vi "readFromXML.vi"(8 "error in (no error)":errorcluster, 10 "XML in":string, 11 "TCSCommand in":refnum<class "TCSCommand.lvclass">) -> (0 "error out":errorcluster, 3 "TCSCommand out":refnum<class "TCSCommand.lvclass">)   [LabVIEW 2014, in "TCSDataDefinitions.lvlib" / "TCSCommand.lvlib" / "TCSCommand.lvclass"]
uses:
  TCSCommand.lvclass
  TCSCommand.lvclass/TCSCommand.ctl
  <userlib>/Common/XML/XMLParser/XMLParser.lvclass
panel:
  out "tcsErrorResponse":errorcluster
  out "commandID":u32
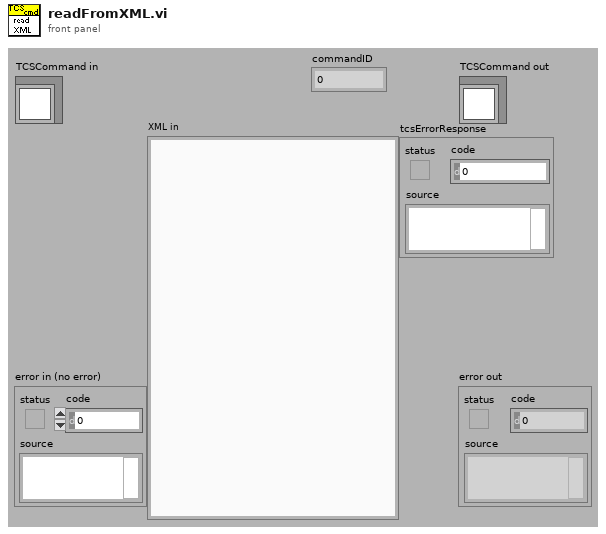
[diagram p1: front panel]
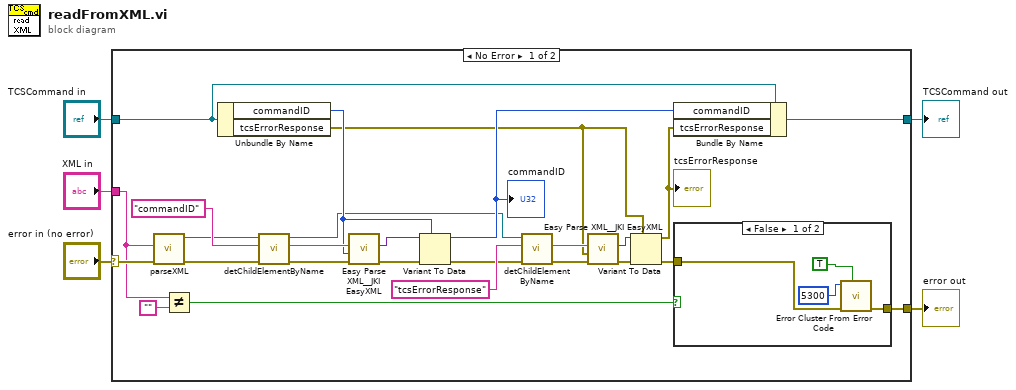
[diagram p0: block diagram]
diagram:
  n1 = case shown="No Error" "error in (no error)" {
    selector: "error in (no error)" -> [w29 w38]
    tunnel: [w10 w38] -> w4
    tunnel: [w15 w37] -> w2
    tunnel: "TCSCommand in" -> [w11 w37]
    tunnel: "XML in" -> [w9 _]
    frame No Error {
      n2 = call <userlib>:"parseXML.vi"("error in (no error)"=w29, "XMLString in"=w9) -> ("error out"=w13:errorcluster, "Element out"=w7:refnum<class "XMLParser.lvclass">)  [unwired: 8 in]
      n3 = Not Equal?(x=w9, y="") -> (x != y?=w30:bool)
      n4 = Unbundle By Name(w11) -> ("commandID"=w21:u32, "tcsErrorResponse"=w12:errorcluster)
      n5 = call <userlib>:"detChildElementByName.vi"("error in (no error)"=w13, "childName"="commandID" ("ChildName"), "Element in"=w7) -> ("error out"=w22:errorcluster, "childXML"=w26:string, "Element out"=w6:refnum<class "XMLParser.lvclass">)  [unwired: 5 in, 1 out]
      n6 = call <vilib>:"Easy Parse XML__JKI EasyXML.vi"("error in (no error)"=w22, "LabVIEW Data (Type)"=w21, "XML String"=w26) -> ("error out"=w23:errorcluster, "LabVIEW Data"=w24:variant)  [unwired: 7 in]
      n7 = Variant To Data(error in=w23, type=w21, Variant=w24) -> (data=w20:u32, error out=w19:errorcluster)
      "commandID" <- w20
      n8 = call <userlib>:"detChildElementByName.vi"("error in (no error)"=w19, "childName"="tcsErrorResponse" ("ChildName"), "Element in"=w6) -> ("error out"=w18:errorcluster, "childXML"=w25:string)  [unwired: 5 in, 2 out]
      n9 = call <vilib>:"Easy Parse XML__JKI EasyXML.vi"("error in (no error)"=w18, "LabVIEW Data (Type)"=w12, "XML String"=w25) -> ("error out"=w14:errorcluster, "LabVIEW Data"=w17:variant)  [unwired: 7 in]
      n10 = Variant To Data(error in=w14, type=w12, Variant=w17) -> (data=w16:errorcluster, error out=w8:errorcluster)
      "tcsErrorResponse" <- w16
      n11 = Bundle By Name(cluster=w11, "commandID"=w20, "tcsErrorResponse"=w16) -> (w15:refnum<class "TCSCommand.lvclass">)
      n12 = case shown="False" w30 {
        tunnel: [w33 w36] -> w10
        tunnel: w8 -> [w34 w36]
        frame False {
          n13 = call <vilib>:"Error Cluster From Error Code.vi"("show call chain? (False)"=TRUE, "error in (no error)"=w34, "error code (0)"=5300 ("code")) -> ("error out"=w33:errorcluster)  [unwired: 6 in]
        }
        frame True {
        }
      }
    }
    frame Error {
    }
  }
  "error out" <- w4
  "TCSCommand out" <- w2
